vi "Excess-64-Byte-Array-to-Real.vi"(11 "Byte array (4 or 8 bytes)":u8[](array[numeric]) format="%08b") -> (3 "Real Number":dbl)   [LabVIEW 2019]
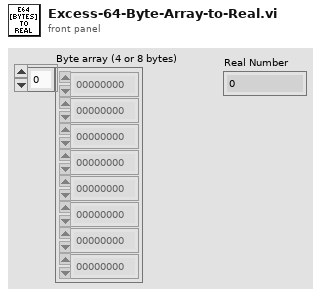
[diagram p1: front panel]
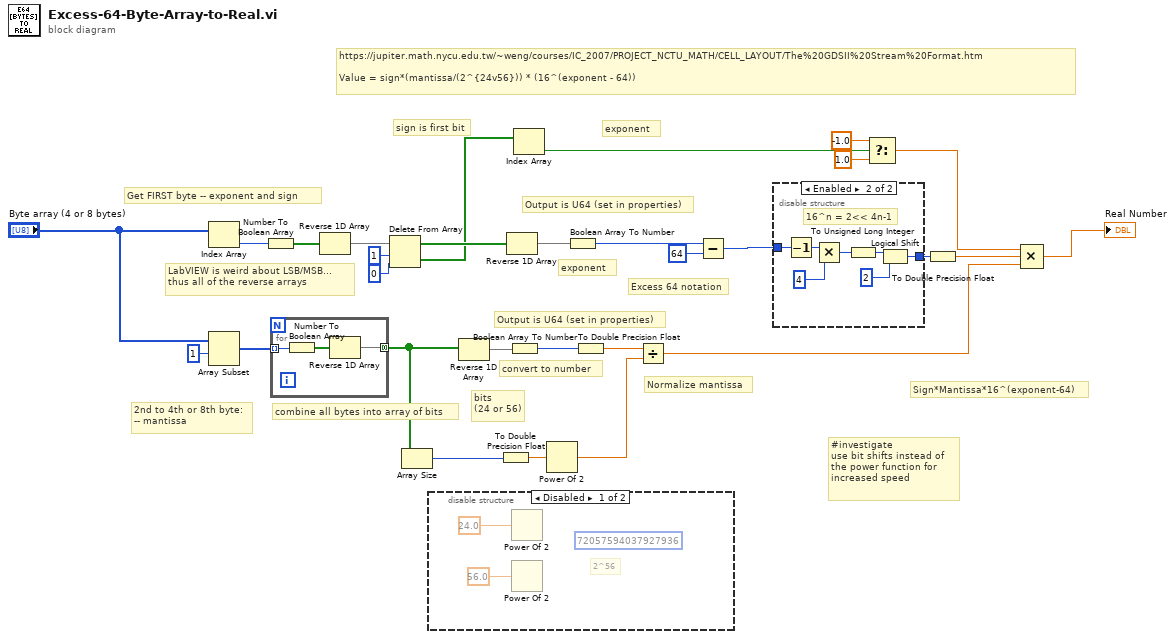
[diagram p0: block diagram]
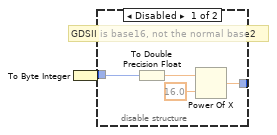
[diagram p2: hidden frame]
diagram:
  # "#investigate\nuse bit shifts instead of the power function for increased speed"
  # "exponent"
  # "bits\n(24 or 56)"
  # "Output is U64 (set in properties)"
  # "https://jupiter.math.nycu.edu.tw/~weng/courses/IC_2007/PROJECT_NCTU_MATH/CELL_LAYOUT/The%20GDSII%20Stream%20Format.htm\n\nValue = sign*(mantissa/(2^{24v56})) * (16^(exponent - 64))"
  # "combine all bytes into array of bits"
  # "LabVIEW is weird about LSB/MSB... thus all of the reverse arrays"
  # "2nd to 4th or 8th byte:\n-- mantissa"
  # "Sign*Mantissa*16^(exponent-64)"
  # "Excess 64 notation"
  # "convert to number"
  # "Normalize mantissa"
  # "exponent"
  # "sign is first bit"
  # "Get FIRST byte -- exponent and sign"
  # "Output is U64 (set in properties)"
  n1 = Index Array(array="Byte array (4 or 8 bytes)") -> (element=w12:u8)  [unwired: 1 in]
  n2 = Array Subset(array="Byte array (4 or 8 bytes)", index=1) -> (w19:u8[])  [unwired: 1 in]
  n3 = Number To Boolean Array(number=w12) -> (Boolean array=w18:bool[])
  n4 = for {
    tunnel: w19 -> [w32] mode=indexing
    tunnel: [w30] -> w13 mode=concatenating
    n5 = Number To Boolean Array(number=w32) -> (Boolean array=w31:bool[])
    n6 = Reverse 1D Array(array=w31) -> (reversed array=w30:bool[])
  }
  n7 = Reverse 1D Array(array=w18) -> (reversed array=w16:bool[])
  n8 = Delete From Array(array=w16, length=1, index=0) -> (deleted portion=w15:bool[], array with subset deleted=w22:bool[])
  n9 = Array Size(array=w13) -> (size(s)=w14:i32)
  n10 = disable-structure shown="Disabled" {
    frame Disabled {
      (unwired) u64 72057594037927936
      # "2^56"
      n11 = Power Of 2(x=24.0) -> ()  [unwired: 1 out]
      n12 = Power Of 2(x=56.0) -> ()  [unwired: 1 out]
    }
    frame Enabled {
    }
  }
  n13 = Reverse 1D Array(array=w13) -> (reversed array=w24:bool[])
  n14 = To Double Precision Float(number=w14) -> (double precision float=w4:dbl)
  n15 = Reverse 1D Array(array=w22) -> (reversed array=w29:bool[])
  n16 = Boolean Array To Number(Boolean array=w24) -> (number=w25:u64)
  n17 = Index Array(array=w15) -> (element=w9:bool)  [unwired: 1 in]
  n18 = Power Of 2(x=w4) -> (2^x=w20:dbl)
  n19 = Boolean Array To Number(Boolean array=w29) -> (number=w26:u64)
  n20 = To Double Precision Float(number=w25) -> (double precision float=w3:dbl)
  n21 = Divide(x=w3, y=w20) -> (x/y=w10:dbl)
  n22 = Subtract(x=w26, y=u64 64) -> (x-y=w28:u64)
  n23 = disable-structure shown="Enabled" {
    disable-tunnel: w28 -> [w38 w46]
    disable-tunnel: [w35 w42] -> w2
    frame Disabled {
      # "GDSII is base16, not the normal base2"
      n24 = To Byte Integer(number=w38) -> (8bit integer=w36:i8)
      n25 = To Double Precision Float(number=w36) -> (double precision float=w39:dbl)
      n26 = Power Of X(1:16.0 ("x"), 2:w39) -> (0:w35:dbl)
    }
    frame Enabled {
      # "16^n = 2<< 4n-1"
      n27 = Decrement(x=w46) -> (x-1=w45:u64)
      n28 = Multiply(x=w45, y=u64 4) -> (x*y=w43:u64)
      n29 = To Unsigned Long Integer(number=w43) -> (unsigned 32bit integer=w41:u32)
      n30 = Logical Shift(y=w41, x=u32 2) -> (x << y=w42:u32)
    }
  }
  n31 = Select(t=-1.0, s=w9, f=1.0) -> (s? t:f=w6:dbl)
  n32 = To Double Precision Float(number=w2) -> (double precision float=w1:dbl)
  n33 = Compound Arithmetic op=MULTIPLY(w6, w1, w10) -> (→"Real Number":dbl)
